vi "XY Chart Buffer.vi"(8 "clear first (no:F)":bool, 9 "chart length (points)":i32=100, 10 "new point":cluster{"x":dbl, "y":dbl} {"y" format="%.2f"; "x" format="%.2f"}) -> (3 "XY chart data":cluster{"x":dbl, "y":dbl}[](array[cluster]) {"y" format="%.2f"; "x" format="%.2f"})   [LabVIEW 2009]
doc: "This reentrant VI uses an XY graph to mimic the behavior of an XY chart, in that it plots a stipulated amount of the most recently acquired data points. The chart data is stored in a static local variable of the output XY chart indicator.\n\nBecause the VI has been marked reentrant (in VI setup), you can make multiple parallel calls to the VI without confusing the memory. Use the new points array input to supply multiple points at once, or leave the array unwired (empty) and use the new point cluster input to supply one point at a time. If the locally stored chart array is not equal to chart length, it is expanded to that length by replicating the most recently acquired point. Data in excess of the history length is discarded. Set clear first to clear the chart history before processing the new points."
panel:
  in  "Case Constant\n(See Context Help)":bool=TRUE
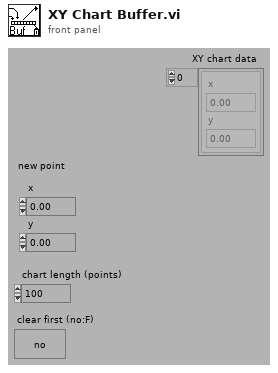
[diagram p1: front panel]
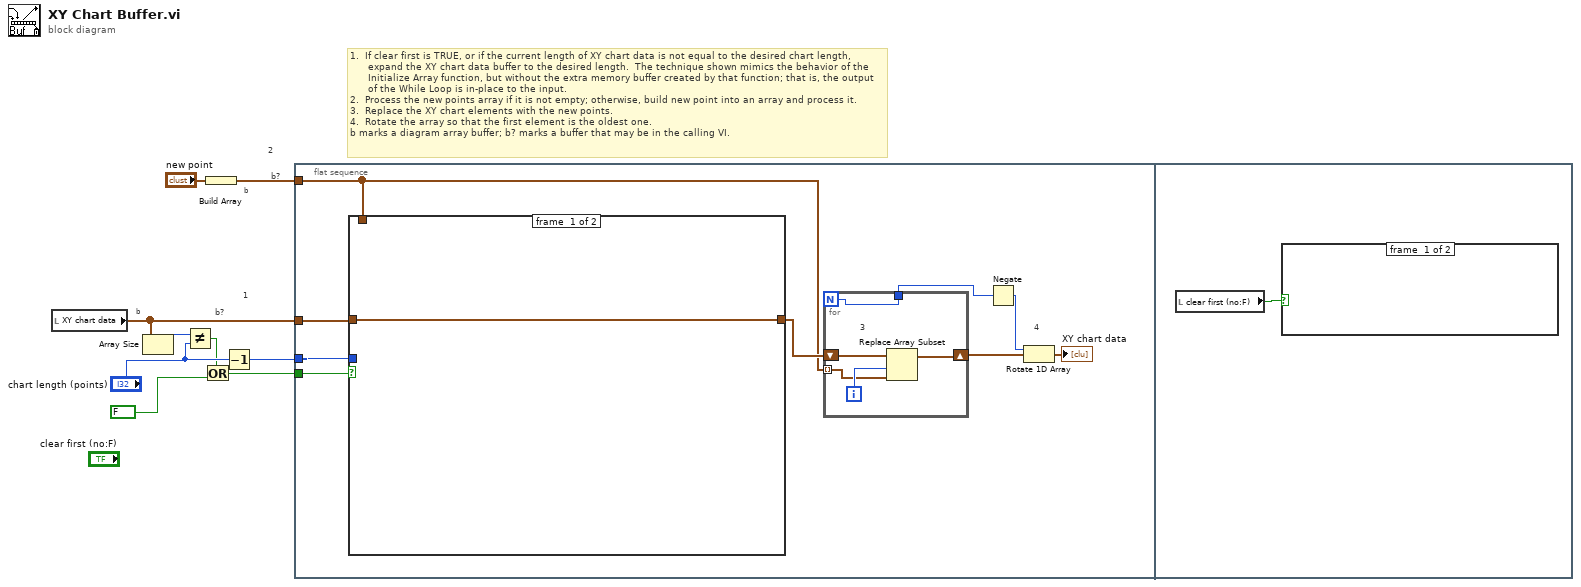
[diagram p0: block diagram]
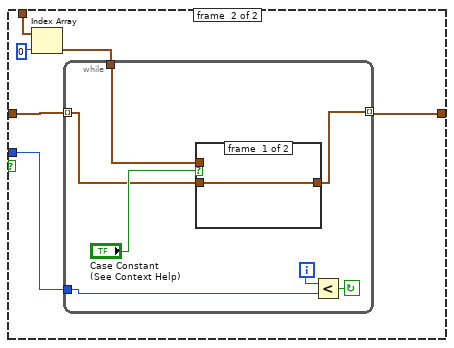
[diagram p2: hidden frame]
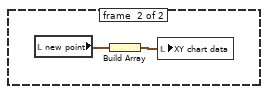
[diagram p4: hidden frame]
diagram:
  # "1.  If clear first is TRUE, or if the current length of XY chart data is not equal to the desired chart length,\n      expand the XY chart data buffer to the desired length.  The technique shown mimics the behavior of the\n      Initialize Array function, but without the extra memory buffer created by that function; that is, the output\n      of the While Loop is in-place to the input.\n2.  Process the new points array if it is not empty; otherwise, build new point into an array and process it.\n3.  Replace the XY chart elements with the new points.  \n4.  Rotate the array so that the first element is the oldest one.\nb marks a diagram array buffer; b? marks a buffer that may be in the calling VI."
  # "b"
  # "2"
  # "1"
  # "b?"
  # "b"
  # "b?"
  n1 = local read "XY chart data"() -> (w3:cluster{"x":dbl, "y":dbl}[])
  n2 = Array Size(array=w3) -> (size(s)=w7:i32)
  n3 = Not Equal?(x=w7, y="chart length (points)") -> (x != y?=w6:bool)
  n4 = Or(x=w6, y=FALSE) -> (x .or. y?=w5:bool)
  n5 = Build Array("new point") -> (w2:cluster{"x":dbl, "y":dbl}[])
  n6 = Decrement(x="chart length (points)") -> (x-1=w4:i32)
  n7 = flat-sequence {
    tunnel: w5 -> [w14]
    tunnel: w4 -> [w13]
    tunnel: w3 -> [w11]
    tunnel: w2 -> [w10]
    frame #0 {
      # "4"
      n8 = case shown="True" w14 {
        tunnel: [w19 w20] -> w16
        tunnel: w13 -> [_ w24]
        tunnel: w11 -> [w19 w25]
        tunnel: w10 -> [_ w22]
        frame #0 {
        }
        frame #1 {
          n9 = Index Array(array=w22, index=0) -> (element=w21:cluster{"x":dbl, "y":dbl})
          n10 = while {
            tunnel: [w28] -> w20 mode=indexing
            tunnel: w21 -> [w26]
            tunnel: w24 -> [w32]
            tunnel: w25 -> [w27] mode=indexing
            i -> [w31]
            stop <- w30 continue-if-true
            n11 = case shown="False" "Case Constant\n(See Context Help)" {
              tunnel: [w33 w34] -> w28
              tunnel: w27 -> [w33 _]
              tunnel: w26 -> [_ w34]
              frame #0 {
              }
              frame #1 {
              }
            }
            n12 = Less?(x=w31, y=w32) -> (x < y?=w30:bool)
          }
        }
      }
      n13 = for {
        N -> [w36]
        shift-right: [w39] -> w17
        shift-left: w16 -> [w37]
        tunnel: w10 -> [w35] mode=indexing
        tunnel: [w36] -> w15
        i -> [w38]
        # "3"
        n14 = Replace Array Subset(array=w37, new element=w35, index=w38) -> (w39:cluster{"x":dbl, "y":dbl}[])
      }
      n15 = Negate(x=w15) -> (-x=w18:i32)
      n16 = Rotate 1D Array(1:w17, 2:w18) -> (0:→"XY chart data":cluster{"x":dbl, "y":dbl}[])
    }
    frame #1 {
      n17 = local read "clear first (no:F)"() -> (w40:bool)
      n18 = case shown="True" w40 {
        frame #0 {
        }
        frame #1 {
          n19 = local read "new point"() -> (w42:cluster{"x":dbl, "y":dbl})
          n20 = Build Array(w42) -> (w41:cluster{"x":dbl, "y":dbl}[])
          n21 = local write "XY chart data"(w41) -> ()
        }
      }
    }
  }
